vi "test Estimate All Positions New.vi"(8 "error in (no error)":errorcluster, 11 "TestCase in":refnum<class "Position Estimation Tests.lvclass">) -> (0 "error out":errorcluster, 3 "TestCase out":refnum<class "Position Estimation Tests.lvclass">)   [LabVIEW 2014, in "Position Estimation Tests.lvclass"]
uses:
  Position Estimation Tests.lvclass
  SPLAT/Anchor/Anchor.lvclass
  <vilib>/addons/_JKI Toolkits/VI Tester/TestCase.llb/TestCase.lvclass
  SPLAT/Position.lvclass
  SPLAT/Tag.lvclass
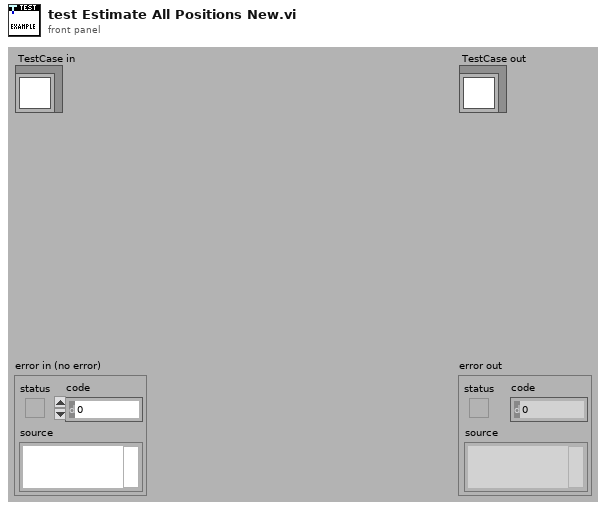
[diagram p1: front panel]
types:
  T1 = cluster{"tagID":dbl, "X":dbl, "Y":dbl, "anchorIDDistanceCluster":cluster{"anchorIDArray":dbl[], "anchorDistanceArray":dbl[]}}
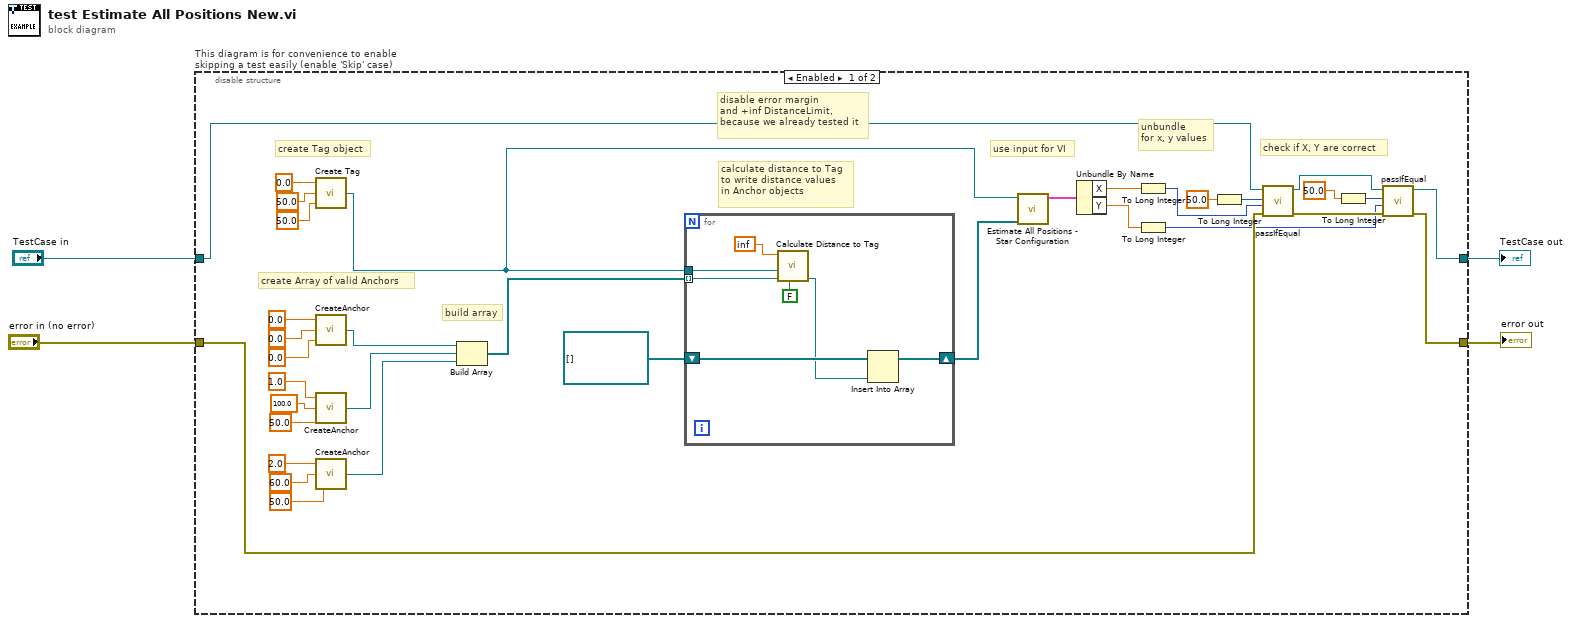
[diagram p0: block diagram]
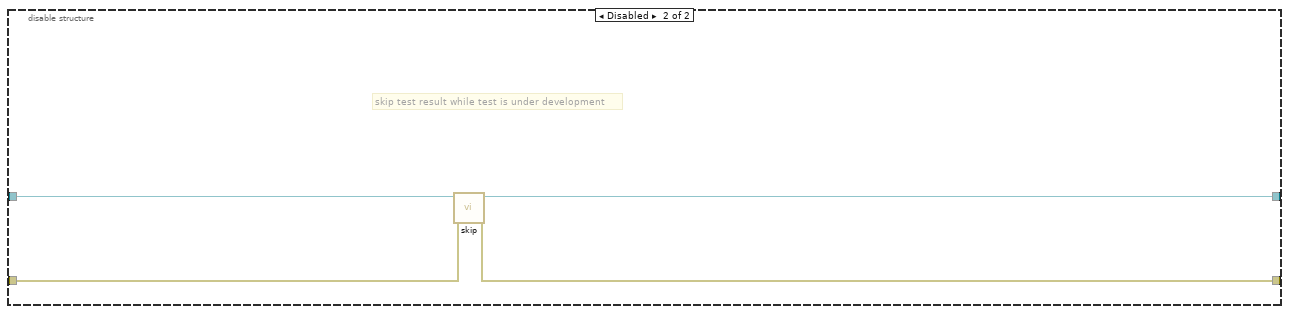
[diagram p2: hidden frame]
diagram:
  n1 = disable-structure "This diagram is for convenience to enable skipping a test easily (enable 'Skip' case)" shown="Enabled" {
    disable-tunnel: "TestCase in" -> [w18 w49]
    disable-tunnel: [w17 w47] -> w1
    disable-tunnel: [w14 w48] -> w3
    disable-tunnel: "error in (no error)" -> [w16 w46]
    frame Enabled {
      # "unbundle\nfor x, y values"
      # "disable error margin\nand +inf DistanceLimit,\nbecause we already tested it"
      # "build array"
      # "calculate distance to Tag\nto write distance values\nin Anchor objects"
      # "check if X, Y are correct"
      # "use input for VI"
      # "create Array of valid Anchors"
      # "create Tag object"
      n2 = call "Create Tag.vi"("TagY"=50.0, "TagX"=50.0, "TagID"=0.0) -> ("Tag Out"=w21:refnum<class "Tag.lvclass">)
      n3 = call "CreateAnchor.vi"("Anchor Y"=0.0, "Anchor X"=0.0, "Anchor ID"=0.0) -> ("Anchor Out"=w26:refnum<class "Anchor.lvclass">)
      n4 = call "CreateAnchor.vi"("Anchor Y"=50.0, "Anchor X"=100.0, "Anchor ID"=1.0) -> ("Anchor Out"=w25:refnum<class "Anchor.lvclass">)
      n5 = call "CreateAnchor.vi"("Anchor Y"=50.0, "Anchor X"=60.0, "Anchor ID"=2.0) -> ("Anchor Out"=w24:refnum<class "Anchor.lvclass">)
      n6 = Build Array(w26, w25, w24) -> (w23:refnum<class "Anchor.lvclass">[])
      n7 = for {
        tunnel: w23 -> [w43] mode=indexing
        tunnel: w21 -> [w42]
        shift-right: [w39] -> w20
        shift-left: refnum<class "Anchor.lvclass">[] [] -> [w41]
        n8 = call "Calculate Distance to Tag.vi"("Enable error margin"=FALSE, "Anchor.lvclass In"=w43, "Tag.lvclass"=w42, "DistanceLimit"=inf) -> ("Anchor out"=w40:refnum<class "Anchor.lvclass">)  [unwired: 6 in, 1 out]
        n9 = Insert Into Array(array=w41, new element=w40) -> (w39:refnum<class "Anchor.lvclass">[])  [unwired: 1 in]
      }
      n10 = call "Estimate All Positions - Star Configuration.vi"("Input AnchorArray"=w20, "Tag.lvclass"=w21) -> ("PositionCluster [tagID, x, y, anchorID, distances]"=w19:T1)  [unwired: 7 in, 2 out]
      n11 = Unbundle By Name(w19) -> ("X"=w10:dbl, "Y"=w13:dbl)
      n12 = To Long Integer(number=w10) -> (32bit integer=w9:i32)
      n13 = To Long Integer(number=w13) -> (32bit integer=w5:i32)
      n14 = To Long Integer(number=50.0) -> (32bit integer=w7:i32)
      n15 = call-dynamic "passIfEqual.vi"("error in (no error)"=w16, "y"=w9, "x"=w7, "TestCase in"=w18) -> ("error out"=w15:errorcluster, "TestCase out"=w6:refnum<class "Position Estimation Tests.lvclass">)  [unwired: 6 in]
      n16 = To Long Integer(number=50.0) -> (32bit integer=w11:i32)
      n17 = call-dynamic "passIfEqual.vi"("error in (no error)"=w15, "y"=w5, "x"=w11, "TestCase in"=w6) -> ("error out"=w14:errorcluster, "TestCase out"=w17:refnum<class "Position Estimation Tests.lvclass">)  [unwired: 6 in]
    }
    frame Disabled {
      # "skip test result while test is under development"
      n18 = call <vilib>:"skip.vi"("error in (no error)"=w46, "TestCase in"=w49) -> ("error out"=w48:errorcluster, "TestCase out"=w47:refnum<class "Position Estimation Tests.lvclass">)  [unwired: 8 in]
    }
  }
  "error out" <- w3
  "TestCase out" <- w1
